vi "Check Level Limit Range.vi"(0 "Intrument Handle[]":refnum<k15>, 5 "Source Mode":T1 items=["DC Voltage", "DC Current"], 7 "Channel Name":string, 11 "error in (no error)":errorcluster) -> (8 "Error from limit":errorcluster, 15 "Error from level":errorcluster)   [LabVIEW 2024, in "devicePowerSequencerCoreLogic.lvlib"]
uses:
  devicePowerSequencerCoreLogic.lvlib
  controls/Source Mode.ctl
  Device Power Sequencer.lvlib
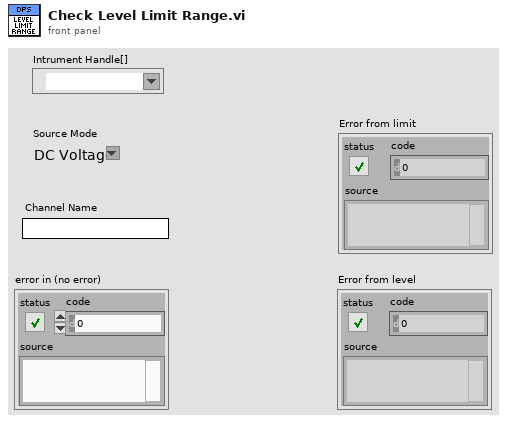
[diagram p1: front panel]
types:
  T1 = typedef "Device Power Sequencer.lvlib/Source Mode.ctl" = i32
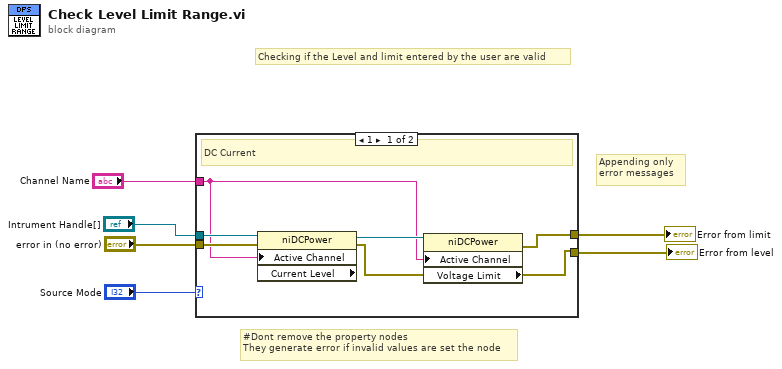
[diagram p0: block diagram]
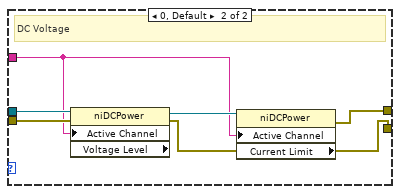
[diagram p2: hidden frame]
diagram:
  # "#Dont remove the property nodes\nThey generate error if invalid values are set the node"
  # "Checking if the Level and limit entered by the user are valid"
  # "Appending only\nerror messages"
  n1 = case shown="1" "Source Mode" {
    tunnel: "error in (no error)" -> [w12 w18]
    tunnel: "Intrument Handle[]" -> [w11 w17]
    tunnel: [w8 w14] -> w2
    tunnel: [w9 w15] -> w3
    tunnel: "Channel Name" -> [w7 w13]
    frame 1 {
      # "DC Current"
      n2 = property class="niDCPower" props=["Active Channel", "Current Level"](reference=w11, error in=w12, "Active Channel"=w7) -> (reference out=w10:refnum<k15>, error out=w8:errorcluster)  [unwired: 1 out]
      n3 = property class="niDCPower" props=["Active Channel", "Voltage Limit"](reference=w10, "Active Channel"=w7) -> (error out=w9:errorcluster)  [unwired: 1 in, 2 out]
    }
    frame 0, Default {
      # "DC Voltage"
      n4 = property class="niDCPower" props=["Active Channel", "Voltage Level"](reference=w17, error in=w18, "Active Channel"=w13) -> (reference out=w16:refnum<k15>, error out=w14:errorcluster)  [unwired: 1 out]
      n5 = property class="niDCPower" props=["Active Channel", "Current Limit"](reference=w16, "Active Channel"=w13) -> (error out=w15:errorcluster)  [unwired: 1 in, 2 out]
    }
  }
  "Error from level" <- w2
  "Error from limit" <- w3
